vi "Shooter_WinchNoPID.vi"(6 "PickStartPos":dbl, 8 "Winch Pot Location":dbl, 9 "WinchPower":dbl=0.75, 10 "selectedCase":i32, 11 "SetPointArray":dbl[](array[numeric])=[1.0, 2.0, 3.0]) -> (0 "isThere?":bool, 3 "Winch Motor Power Out":dbl)   [LabVIEW 2013]
panel:
  out "Winch Desired Location":dbl
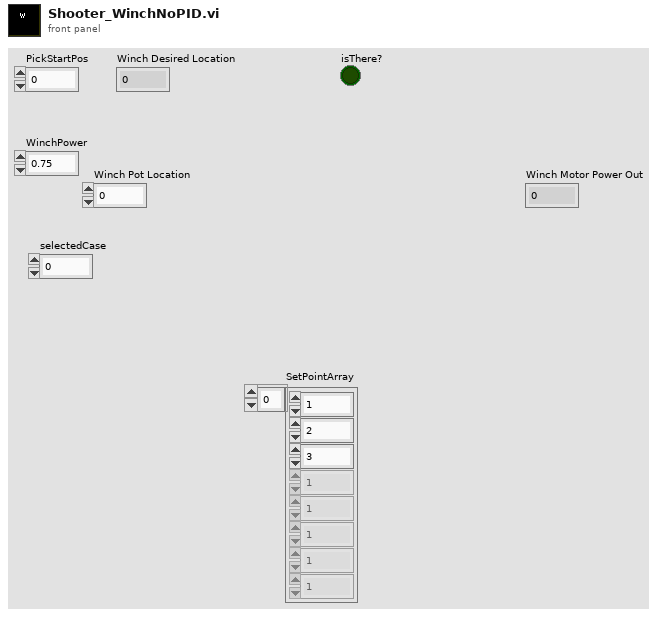
[diagram p1: front panel]
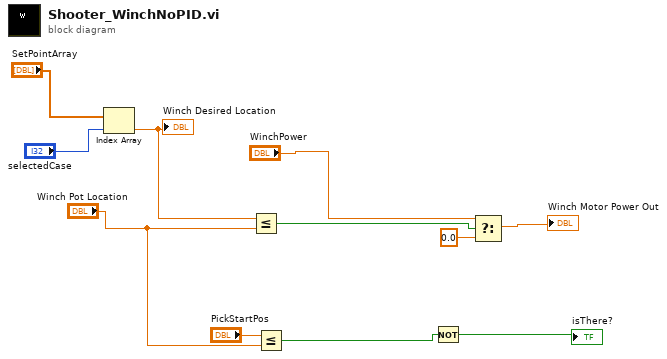
[diagram p0: block diagram]
diagram:
  n1 = Index Array(array="SetPointArray", index="selectedCase") -> (element=w7:dbl)
  "Winch Desired Location" <- w7
  n2 = Less Or Equal?(x=w7, y="Winch Pot Location") -> (x <= y?=w5:bool)
  n3 = Less Or Equal?(x="PickStartPos", y="Winch Pot Location") -> (x <= y?=w3:bool)
  n4 = Not(x=w3) -> (.not. x?=→"isThere?":bool)
  n5 = Select(t="WinchPower", s=w5, f=0.0) -> (s? t:f=→"Winch Motor Power Out":dbl)
